vi "Read ID.vi"(8 "error in (no error)":errorcluster, 11 "Simple ID Mailman in":refnum<class "Simple ID Mailman.lvclass">) -> (0 "error out":errorcluster, 2 "ID":i64, 3 "Simple ID Mailman out":refnum<class "Simple ID Mailman.lvclass">)   [LabVIEW 2024, in "Simple ID Mailman.lvclass"]
uses:
  Simple ID Mailman.lvclass
  Simple ID Mailman.lvclass/Simple ID Mailman.ctl
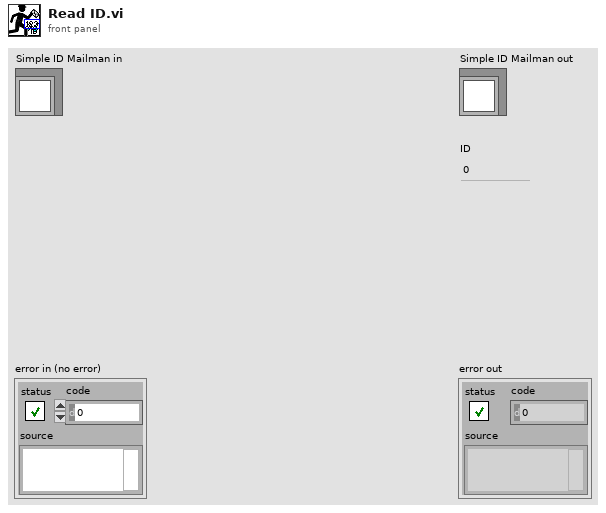
[diagram p1: front panel]
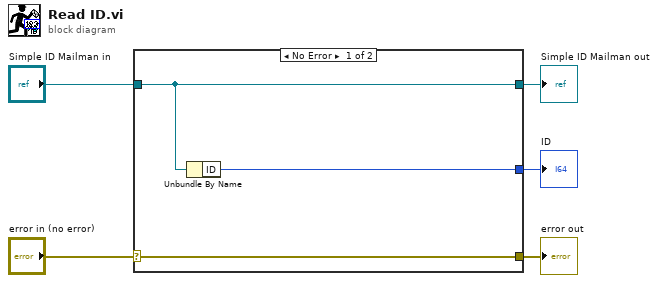
[diagram p0: block diagram]
diagram:
  n1 = case shown="No Error" "error in (no error)" {
    selector: "error in (no error)" -> [w8 w9]
    tunnel: [w8 w9] -> w4
    tunnel: [w7 w10] -> w2
    tunnel: "Simple ID Mailman in" -> [w7 w10]
    tunnel: [w6 _] -> w1
    frame No Error {
      n2 = Unbundle By Name(w7) -> ("ID"=w6:i64)
    }
    frame Error {
    }
  }
  "error out" <- w4
  "Simple ID Mailman out" <- w2
  "ID" <- w1
